vi "StateSelector.vi"(9 "Conditional State":T1, 10 "Default State":T1, 11 "Action Button":bool) -> (3 "Output State":T1)   [LabVIEW 2019]
doc: "This VI checks if action button is pressed, if so then move to its procedure"
uses:
  #typedef_ProgramStates.ctl
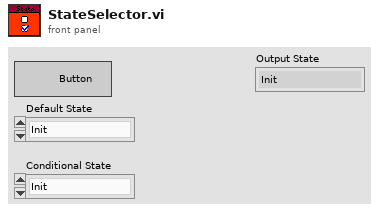
[diagram p1: front panel]
types:
  T1 = typedef "#typedef_ProgramStates.ctl" = enum16{"Init", "Clicking on Piece", "Clicking on Square", "Checking Movement", "Checking King  ", "Checking if Mate", "End"}
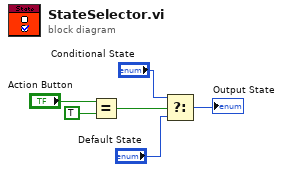
[diagram p0: block diagram]
diagram:
  n1 = Equal?(x="Action Button", y=TRUE) -> (x = y?=w6:bool)
  n2 = Select(t="Conditional State", s=w6, f="Default State") -> (s? t:f=→"Output State":T1)
